vi "About.vi"() -> ()   [LabVIEW 2013, in "Caraya.lvlib" / "Basic Test Manager.lvclass"]
uses:
  Basic Test Manager.lvclass
  Caraya.lvlib
panel:
  out "String":string
types:
  T1 = enum32{"Invalid", "Standard", "Closed", "Hidden", "Minimized", "Maximized"}
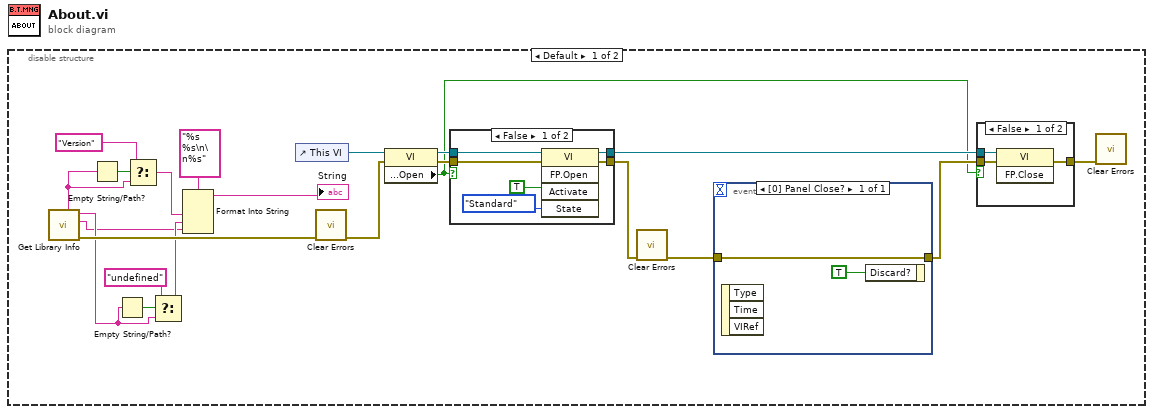
[diagram p0: block diagram]
diagram:
  n1 = disable-structure shown="Default" {
    frame condition #0 (active) {
      n2 = call "Get Library Info.vi"() -> ("error out"=w12:errorcluster, "Copyright"=w1:string, "Version String"=w2:string, "Name"=w8:string)  [unwired: 7 in, 1 out]
      n3 = Empty String/Path?(string/path=w8) -> (empty?=w9:bool)
      n4 = Empty String/Path?(string/path=w2) -> (empty?=w5:bool)
      n5 = Select(t="Version", s=w9, f=w8) -> (s? t:f=w7:string)
      n6 = Select(t="undefined", s=w5, f=w2) -> (s? t:f=w3:string)
      n7 = Format Into String(format string="%s %s\n\n%s", w7, w3, w1) -> (resulting string=→"String":string)  [unwired: 2 in, 1 out]
      n8 = control-ref of="This VI"() -> (w22:refnum<vi>)
      n9 = call <vilib>:"Clear Errors.vi"("error in (no error)"=w12) -> ("error out"=w18:errorcluster)  [unwired: 6 in]
      n10 = property class="VI"(reference=w22, error in=w18) -> (reference out=w20:refnum<vi>, error out=w21:errorcluster, "Front Panel.Open"=w13:bool)
      n11 = case shown="False" w13 {
        tunnel: [w30 w34] -> w19
        tunnel: w21 -> [w29 w34]
        tunnel: w20 -> [w28 w33]
        tunnel: [w27 w33] -> w15
        frame False {
          n12 = invoke class="VI" method="FP.Open"(reference=w28, error in=w29, "Activate"=TRUE, "State"=T1."Standard") -> (reference out=w27:refnum<vi>, error out=w30:errorcluster)  [unwired: 1 in, 3 out]
        }
        frame True {
        }
      }
      n13 = call <vilib>:"Clear Errors.vi"("error in (no error)"=w19) -> ("error out"=w17:errorcluster)  [unwired: 6 in]
      n14 = event shown="[0] Panel Close?" {
        selector: _ -> [_]
        dyn-events: _ -> [_]
        timeout: _ -> [_]
        tunnel: w17 -> [w35]
        tunnel: [w35] -> w14
        event Panel Close? {
          n15 = event-data() -> ()  [unwired: 1 in, 3 out]
          n16 = event-data("Discard?"=TRUE) -> ()  [unwired: 1 in, 1 out]
        }
      }
      n17 = case shown="False" w13 {
        tunnel: [w25 w26] -> w16
        tunnel: w14 -> [w24 w26]
        tunnel: w15 -> [w23 _]
        frame False {
          n18 = invoke class="VI" method="FP.Close"(reference=w23, error in=w24) -> (error out=w25:errorcluster)  [unwired: 1 in, 2 out]
        }
        frame True {
        }
      }
      n19 = call <vilib>:"Clear Errors.vi"("error in (no error)"=w16) -> ()  [unwired: 6 in, 1 out]
    }
    frame condition #1 {
    }
  }
